vi "PULL-REPORTS.vi"() -> ()   [LabVIEW 2012]
panel:
  out "stderr":string
  out "stdout":string
  in  "error out":errorcluster
  in  "2010-2013":bool=TRUE
  in  "2011-2013":bool=TRUE
  in  "2012-2013":bool=TRUE
  # "Copy reports form UGDG Client machine"
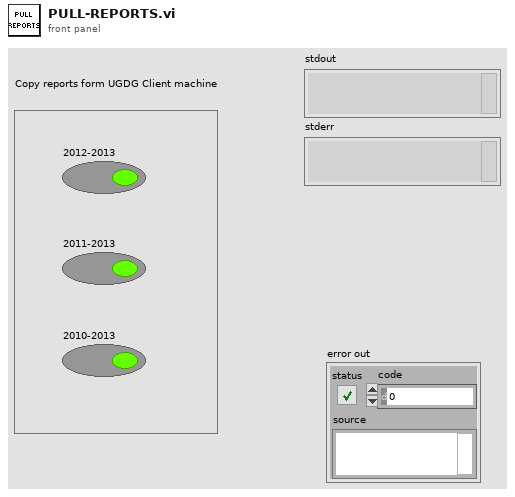
[diagram p1: front panel]
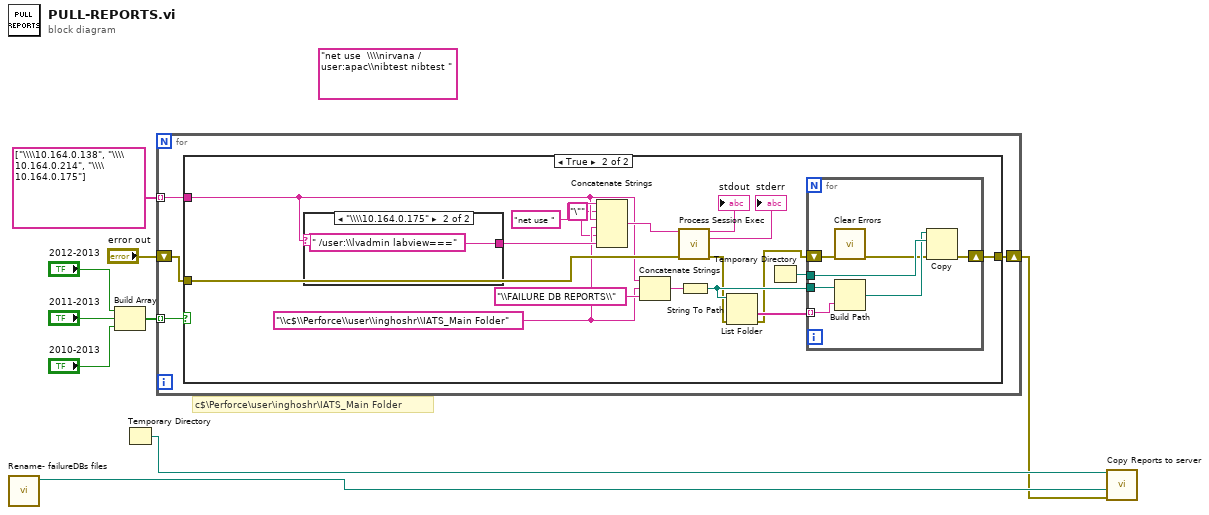
[diagram p0: block diagram]
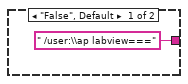
[diagram p3: hidden frame]
diagram:
  (unwired) "net use  \\\\nirvana /user:apac\\nibtest nibtest " ("command line")
  # "c$\\Perforce\\user\\inghoshr\\IATS_Main Folder"
  n1 = call "Rename- failureDBs files.vi"() -> ("Path to copy to!"=w4:path)  [unwired: 11 in]
  n2 = Build Array("2012-2013", "2011-2013", "2010-2013") -> (w7:bool[])
  n3 = Temporary Directory() -> (w3:path)
  n4 = for {
    tunnel: string[] ["\\\\10.164.0.138", "\\\\10.164.0.214", "\\\\10.164.0.175"] -> [w13] mode=indexing
    tunnel: w7 -> [w12] mode=indexing
    shift-right: [w11] -> w1
    shift-left: "error out" -> [w10]
    n5 = case shown="True" w12 {
      tunnel: w13 -> [_ w19]
      tunnel: [w14 w22] -> w11
      tunnel: w10 -> [w14 w21]
      frame False {
      }
      frame True {
        w17 = "\"" ("string")
        w18 = "\\c$\\Perforce\\user\\inghoshr\\IATS_Main Folder" ("string")
        n6 = case shown="\"\\\\\\\\10.164.0.175\"" w19 {
          tunnel: [" /user:\\ap labview===" ("string") " /user:\\lvadmin labview===" ("string")] -> w25
          frame "False", Default {
          }
          frame "\\\\10.164.0.175" {
          }
        }
        n7 = Concatenate Strings("net use " ("string"), w17, w19, w18, w17, w25) -> (w31:string)
        n8 = Concatenate Strings(w19, w18, "\\FAILURE DB REPORTS\\" ("name or relative path")) -> (w29:string)
        n9 = call "Process Session Exec.vi"("command line"=w31, "error in (no error)"=w21) -> ("stdout"=→"stdout":string, "stderr"=→"stderr":string, "error out"=w24:errorcluster)  [unwired: 9 in, 2 out]
        n10 = String To Path(string=w29) -> (path=w27:path)
        n11 = List Folder(path=w27, error in=w24) -> (folder names=w26:string[], error out=w23:errorcluster)  [unwired: 2 in, 2 out]
        n12 = Temporary Directory() -> (w28:path)
        n13 = for {
          tunnel: w28 -> [w40]
          tunnel: w27 -> [w39]
          tunnel: w26 -> [w38] mode=indexing
          shift-right: [w36] -> w22
          shift-left: w23 -> [w35]
          n14 = call <vilib>:"Clear Errors.vi"("error in (no error)"=w35) -> ("error out"=w34:errorcluster)  [unwired: 6 in]
          n15 = Build Path(base path=w39, name or relative path=w38) -> (appended path=w37:path)
          n16 = Copy(8:w34, 10:w40, 11:w37) -> (0:w36:errorcluster)  [unwired: 2 in, 2 out]
        }
      }
    }
  }
  n17 = call "Copy Reports to server.vi"("error in (no error)"=w1, "Path to copy to?"=w4, "Path to copy from?"=w3) -> ()  [unwired: 8 in, 1 out]
